vi "_save_csv_EVM_Only.vi"(7 "delimiter (\\t)":string="SingleCh_", 11 "Data":dbl[][](array[numeric])) -> (3 "FileName":string)   [LabVIEW 2023]
uses:
  <vilib>/Utility/file.llb/Write Delimited Spreadsheet (string).vi
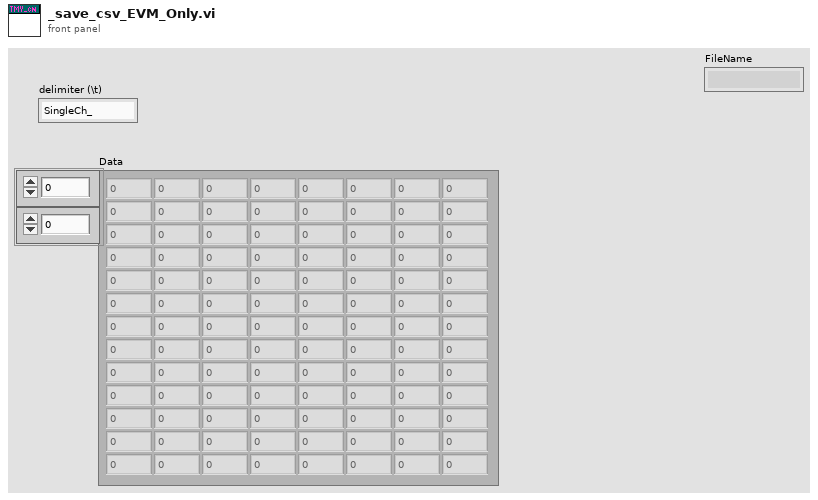
[diagram p1: front panel]
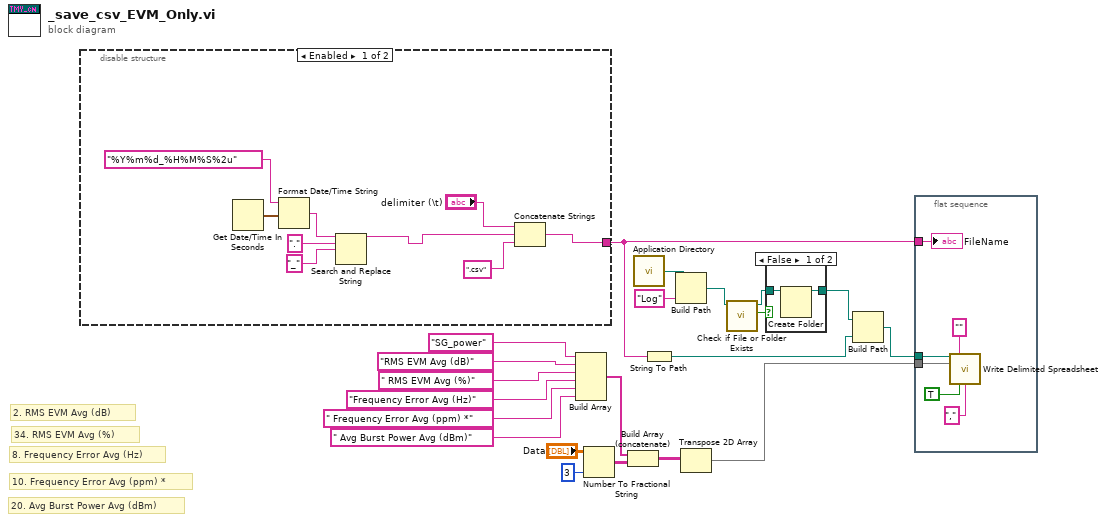
[diagram p0: block diagram]
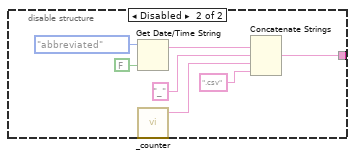
[diagram p3: hidden frame]
diagram:
  # "34. RMS EVM Avg (%)"
  # "20. Avg Burst Power Avg (dBm)"
  # "10. Frequency Error Avg (ppm) *"
  # "2. RMS EVM Avg (dB)"
  # "8. Frequency Error Avg (Hz)"
  n1 = disable-structure shown="Enabled" {
    disable-tunnel: [w29 w31] -> w18
    frame Enabled {
      n2 = Get Date/Time In Seconds() -> (seconds since 1Jan1904=w27:timestamp)
      n3 = Format Date/Time String(time format string (%c)="%Y%m%d_%H%M%S%2u", seconds (now)=w27) -> (date/time string=w25:string)  [unwired: 1 in]
      n4 = Search and Replace String(input string=w25, search string=".", replace string="_") -> (result string=w22:string)  [unwired: 5 in, 3 out]
      n5 = Concatenate Strings("delimiter (\\t)", w22, ".csv" ("delimiter (\\t)")) -> (w29:string)
    }
    frame Disabled {
      n6 = Get Date/Time String(date format (0)=enum16{"short", "long", "abbreviated"}."abbreviated", want seconds? (F)=FALSE) -> (date string=w38:string)  [unwired: 1 in, 1 out]
      n7 = call "_counter.vi"() -> ("out_count"=w32:string)  [unwired: 5 in]
      n8 = Concatenate Strings(w38, "_" ("delimiter (\\t)"), w32, ".csv" ("delimiter (\\t)")) -> (w31:string, w33:string)
    }
  }
  n9 = Build Array("SG_power", "RMS EVM Avg (dB)", " RMS EVM Avg (%)", "Frequency Error Avg (Hz)", " Frequency Error Avg (ppm) *", " Avg Burst Power Avg (dBm)") -> (w7:string[])
  n10 = Number To Fractional String(number="Data", precision (6)=i16 3) -> (F-format string=w8:string[][])  [unwired: 2 in]
  n11 = Build Array (concatenate)(w7, w8) -> (w6:string[][])
  n12 = call <vilib>:"Application Directory.vi"() -> ("Application Directory"=w17:path)
  n13 = String To Path(string=w18) -> (path=w20:path)
  n14 = Build Path(base path=w17, name or relative path="Log") -> (appended path=w14:path)
  n15 = Transpose 2D Array(2D array=w6) -> (transposed array=w5:string[][])
  n16 = call <vilib>:"Check if File or Folder Exists.vi"("path"=w14) -> ("file or folder exists?"=w16:bool, "dup path"=w15:path)  [unwired: 8 in, 1 out]
  n17 = case shown="False" w16 {
    tunnel: w15 -> [w40 w41]
    tunnel: [w39 w41] -> w13
    frame False {
      n18 = Create Folder(path (use dialog)=w40) -> (created path=w39:path)  [unwired: 2 in, 2 out]
    }
    frame True {
    }
  }
  n19 = Build Path(base path=w13, name or relative path=w20) -> (appended path=w19:path)
  n20 = flat-sequence {
    tunnel: w19 -> [w46]
    tunnel: w18 -> [w44]
    tunnel: w5 -> [w42]
    frame #0 {
      n21 = call-poly <vilib>:"Write Delimited Spreadsheet.vi"("file path (dialog if empty)"=w46, "format (%s)"="" ("format (%.3f)"), "2D data"=w42, "transpose? (no:F)"=TRUE, "delimiter (\\t)"="," ("delimiter (\\t)")) -> ()  [unwired: 9 in, 2 out]
      "FileName" <- w44
    }
  }
